vi "VI Tree.vi"   [LabVIEW 2021, in "Keysight XSAnVMA.lvlib"]
doc: "The VI Tree displays all the user-callable VIs of the instrument driver in an organized table."
uses:
  <instrlib>/Keysight XSAnVMA/Keysight XSAnVMA.lvlib
panel:
  # "XSAnVMA"
  # "1.0.4"
  # "SEE DIAGRAM\nFOR VI Tree"
  # "© Keysight Technologies 2018 - 2019"
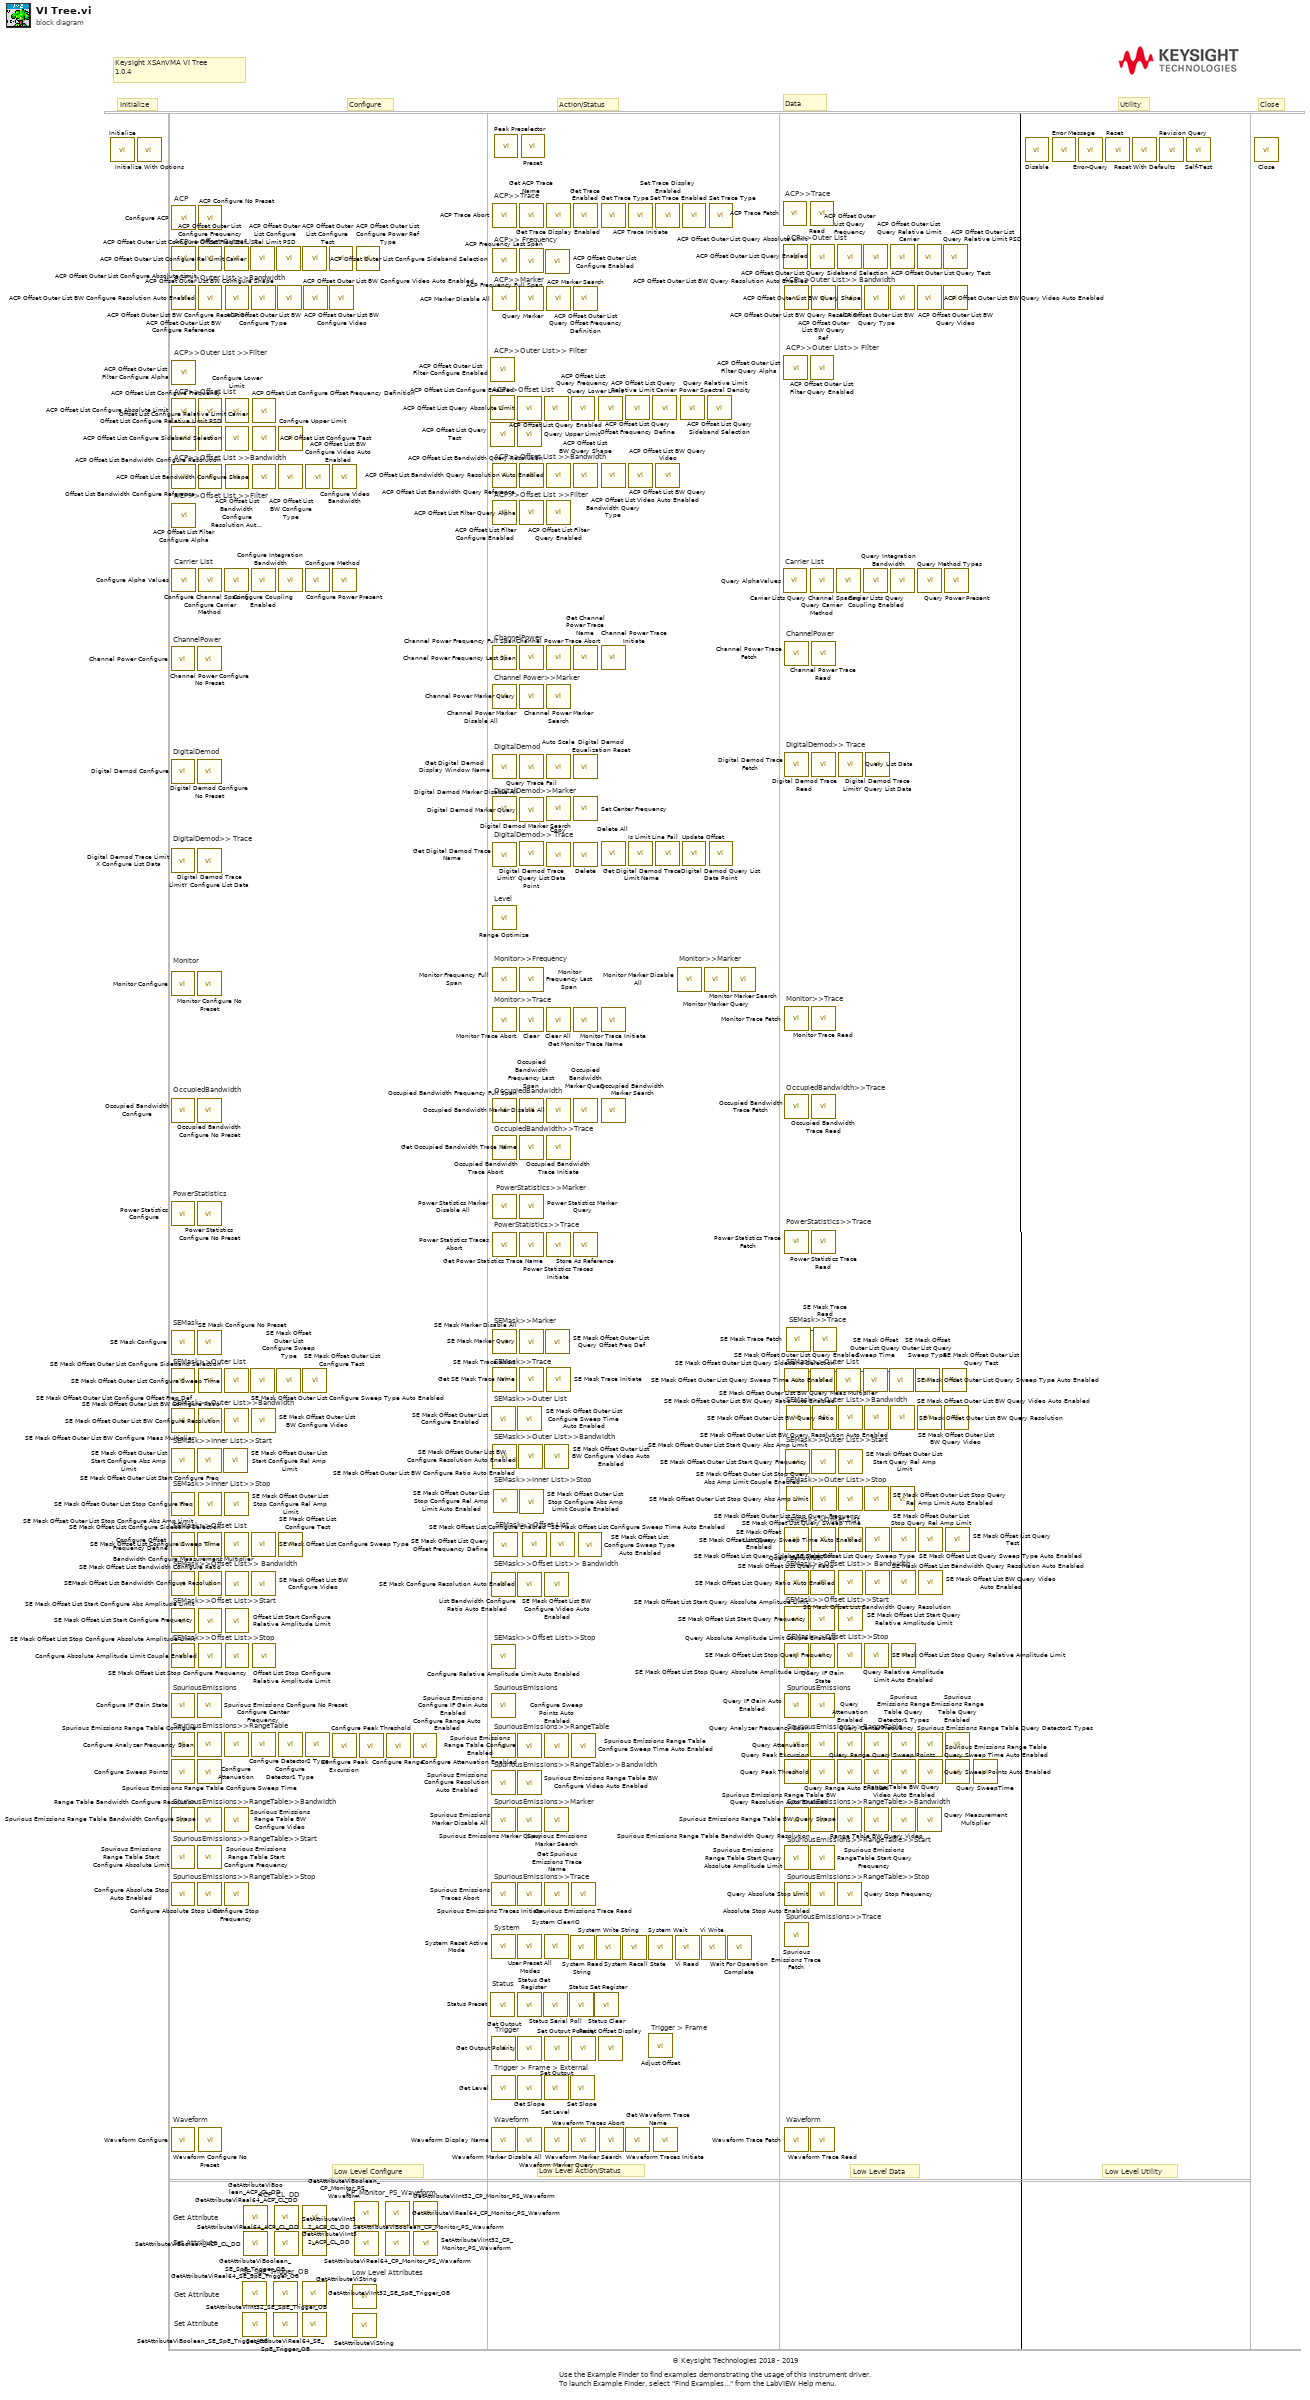
[diagram p0: block diagram]
diagram:
  # "Status"
  # "ACP>>Outer List"
  # "ACP>>Outer List>> Filter"
  # "ACP>>Outer List>> Bandwidth"
  # "Trigger > Frame > External"
  # "Trigger > Frame"
  # "Low Level Attributes"
  # "SE_SpE_Trigger_OB"
  # "CP_Monitor_PS_Waveform"
  # "Set Attribute"
  # "Get Attribute"
  # "Set Attribute"
  # "Get Attribute"
  # "ACP_CL_DD"
  # "Waveform"
  # "SpuriousEmissions>>Trace"
  # "SpuriousEmissions>>RangeTable>>Stop"
  # "SEMask>>Trace"
  # "ACP>>Trace"
  # "SpuriousEmissions>>RangeTable>>Bandwidth"
  # "SpuriousEmissions>>RangeTable"
  # "SpuriousEmissions"
  # "SEMask>>Offset List>>Stop"
  # "SEMask>>Offset List>> Bandwidth"
  # "SEMask>>Inner List>>Stop"
  # "SEMask>>Outer List>>Bandwidth"
  # "SEMask>>Outer List"
  # "ACP>>Offset Outer List"
  # "Waveform"
  # "SpuriousEmissions>>Trace"
  # "SpuriousEmissions>>RangeTable>>Stop"
  # "SpuriousEmissions>>RangeTable>>Start"
  # "SpuriousEmissions>>RangeTable>>Start"
  # "SpuriousEmissions>>RangeTable>>Bandwidth"
  # "SpuriousEmissions>>RangeTable>>Bandwidth"
  # "SpuriousEmissions>>RangeTable"
  # "SpuriousEmissions>>RangeTable"
  # "SpuriousEmissions"
  # "SpuriousEmissions>>Marker"
  # "SEMask>>Offset List"
  # "SEMask>>Trace"
  # "SEMask>>Outer List"
  # "SEMask>>Offset List>> Bandwidth"
  # "SEMask>>Offset List>>Stop"
  # "SEMask>>Offset List>>Start"
  # "SEMask>>Offset List>>Stop"
  # "SEMask>>Offset List>>Start"
  # "SEMask>>Offset List>> Bandwidth"
  # "SEMask>>Offset List"
  # "SEMask>>Offset List"
  # "SEMask>>Outer List>>Stop"
  # "SEMask>>Inner List>>Stop"
  # "SEMask>>Outer List>>Start"
  # "SEMask>>Inner List>>Start"
  # "SEMask>>Outer List>>Bandwidth"
  # "SEMask>>Outer List>>Bandwidth"
  # "SEMask>>Outer List"
  # "SEMask>>Marker"
  # "ChannelPower"
  # "Monitor>>Trace"
  # "OccupiedBandwidth>>Trace"
  # "PowerStatistics>>Trace"
  # "PowerStatistics>>Trace"
  # "PowerStatistics>>Marker"
  # "OccupiedBandwidth>>Trace"
  # "OccupiedBandwidth"
  # "Monitor>>Trace"
  # "Monitor>>Marker"
  # "Monitor>>Frequency"
  # "DigitalDemod>> Trace"
  # "DigitalDemod>> Trace"
  # "DigitalDemod>> Trace"
  # "DigitalDemod"
  # "ChannelPower"
  # "ACP>>Offset List >>Filter"
  # "ACP>>Outer List>> Filter"
  # "ACP>>Offset List >>Bandwidth"
  # "ACP>>Offset List"
  # "ACP>>Outer List >>Filter"
  # "ACP>>Outer List >>Bandwidth"
  # "ACP>> Frequency"
  # "Carrier List"
  # "Low Level Utility"
  # "Low Level Configure"
  # "Low Level Action/Status"
  # "Low Level Data"
  # "Action/Status"
  # "Keysight XSAnVMA VI Tree\n1.0.4"
  # "© Keysight Technologies 2018 - 2019"
  # "Close"
  # "Utility"
  # "Data"
  # "Configure"
  # "Initialize"
  # "Use the Example Finder to find examples demonstrating the usage of this instrument driver.\nTo launch Example Finder, select \"Find Examples...\" from the LabVIEW Help menu."
  # "Waveform"
  # "Trigger"
  # "System"
  # "SpuriousEmissions"
  # "SEMask"
  # "PowerStatistics"
  # "OccupiedBandwidth"
  # "Monitor"
  # "Level"
  # "DigitalDemod>>Marker"
  # "DigitalDemod"
  # "Channel Power>>Marker"
  # "ChannelPower"
  # "ACP>>Trace"
  # "ACP>>Offset List >>Filter"
  # "ACP>>Offset List >>Bandwidth"
  # "ACP>>Offset List"
  # "ACP>>Marker"
  # "Carrier List"
  # "ACP"
  n1 = call <instrlib>:"Initialize.vi"() -> ()  [unwired: 10 in, 2 out]
  n2 = call <instrlib>:"Initialize With Options.vi"() -> ()  [unwired: 10 in, 2 out]
  n3 = call <instrlib>:"Channel Power Configure.vi"() -> ()  [unwired: 10 in, 2 out]
  n4 = call <instrlib>:"Digital Demod Configure.vi"() -> ()  [unwired: 10 in, 2 out]
  n5 = call <instrlib>:"Digital Demod Trace Limit X Configure List Data.vi"() -> ()  [unwired: 10 in, 2 out]
  n6 = call <instrlib>:"Monitor Configure.vi"() -> ()  [unwired: 10 in, 2 out]
  n7 = call <instrlib>:"Occupied Bandwidth Configure.vi"() -> ()  [unwired: 10 in, 2 out]
  n8 = call <instrlib>:"Power Statistics Configure.vi"() -> ()  [unwired: 10 in, 2 out]
  n9 = call <instrlib>:"SE Mask Configure.vi"() -> ()  [unwired: 10 in, 2 out]
  n10 = call <instrlib>:"SE Mask Offset Outer List Configure Offset Freq Def.vi"() -> ()  [unwired: 10 in, 2 out]
  n11 = call <instrlib>:"SE Mask Offset Outer List BW Configure Meas Multiplier.vi"() -> ()  [unwired: 10 in, 2 out]
  n12 = call <instrlib>:"SE Mask Offset Outer List Start Configure Abs Amp Limit.vi"() -> ()  [unwired: 10 in, 2 out]
  n13 = call <instrlib>:"SE Mask Offset Outer List Stop Configure Abs Amp Limit.vi"() -> ()  [unwired: 10 in, 2 out]
  n14 = call <instrlib>:"Configure Offset Frequency Define.vi"() -> ()  [unwired: 10 in, 2 out]
  n15 = call <instrlib>:"Bandwidth Configure Measurement Multiplier.vi"() -> ()  [unwired: 10 in, 2 out]
  n16 = call <instrlib>:"SE Mask Offset List Start Configure Abs Amplitude Limit.vi"() -> ()  [unwired: 10 in, 2 out]
  n17 = call <instrlib>:"SE Mask Offset List Stop Configure Absolute Amplitude Limit.vi"() -> ()  [unwired: 10 in, 2 out]
  n18 = call <instrlib>:"Configure IF Gain State.vi"() -> ()  [unwired: 10 in, 2 out]
  n19 = call <instrlib>:"Spurious Emissions Range Table Configure.vi"() -> ()  [unwired: 10 in, 2 out]
  n20 = call <instrlib>:"Configure Sweep Points.vi"() -> ()  [unwired: 10 in, 2 out]
  n21 = call <instrlib>:"Range Table Bandwidth Configure Resolution.vi"() -> ()  [unwired: 10 in, 2 out]
  n22 = call <instrlib>:"Spurious Emissions Range Table Start Configure Absolute Limit.vi"() -> ()  [unwired: 10 in, 2 out]
  n23 = call <instrlib>:"Configure Absolute Stop Auto Enabled.vi"() -> ()  [unwired: 10 in, 2 out]
  n24 = call <instrlib>:"Waveform Configure.vi"() -> ()  [unwired: 10 in, 2 out]
  n25 = call <instrlib>:"Configure ACP.vi"() -> ()  [unwired: 10 in, 2 out]
  n26 = call <instrlib>:"ACP Offset Outer List Configure Absolute Limit.vi"() -> ()  [unwired: 10 in, 2 out]
  n27 = call <instrlib>:"ACP Offset Outer List BW Configure Reference.vi"() -> ()  [unwired: 10 in, 2 out]
  n28 = call <instrlib>:"ACP Offset Outer List Filter Configure Alpha.vi"() -> ()  [unwired: 10 in, 2 out]
  n29 = call <instrlib>:"ACP Offset List Configure Absolute Limit.vi"() -> ()  [unwired: 10 in, 2 out]
  n30 = call <instrlib>:"Offset List Configure Relative Limit Carrier.vi"() -> ()  [unwired: 10 in, 2 out]
  n31 = call <instrlib>:"Offset List Bandwidth Configure Reference.vi"() -> ()  [unwired: 10 in, 2 out]
  n32 = call <instrlib>:"ACP Offset List Filter Configure Alpha.vi"() -> ()  [unwired: 10 in, 2 out]
  n33 = call <instrlib>:"Configure Alpha Values.vi"() -> ()  [unwired: 10 in, 2 out]
  n34 = call <instrlib>:"Channel Power Configure No Preset.vi"() -> ()  [unwired: 10 in, 2 out]
  n35 = call <instrlib>:"Digital Demod Configure No Preset.vi"() -> ()  [unwired: 10 in, 2 out]
  n36 = call <instrlib>:"Digital Demod Trace LimitY Configure List Data.vi"() -> ()  [unwired: 10 in, 2 out]
  n37 = call <instrlib>:"Monitor Configure No Preset.vi"() -> ()  [unwired: 10 in, 2 out]
  n38 = call <instrlib>:"Occupied Bandwidth Configure No Preset.vi"() -> ()  [unwired: 10 in, 2 out]
  n39 = call <instrlib>:"Power Statistics Configure No Preset.vi"() -> ()  [unwired: 10 in, 2 out]
  n40 = call <instrlib>:"SE Mask Configure No Preset.vi"() -> ()  [unwired: 10 in, 2 out]
  n41 = call <instrlib>:"SE Mask Offset Outer List Start Configure Freq.vi"() -> ()  [unwired: 10 in, 2 out]
  n42 = call <instrlib>:"SE Mask Offset List Configure Sideband Selection.vi"() -> ()  [unwired: 10 in, 2 out]
  n43 = call <instrlib>:"Spurious Emissions Configure No Preset.vi"() -> ()  [unwired: 10 in, 2 out]
  n44 = call <instrlib>:"Configure Analyzer Frequency Span.vi"() -> ()  [unwired: 10 in, 2 out]
  n45 = call <instrlib>:"Spurious Emissions Range Table Configure Sweep Time.vi"() -> ()  [unwired: 10 in, 2 out]
  n46 = call <instrlib>:"Spurious Emissions Range Table Bandwidth Configure Shape.vi"() -> ()  [unwired: 10 in, 2 out]
  n47 = call <instrlib>:"Spurious Emissions Range Table Start Configure Frequency.vi"() -> ()  [unwired: 10 in, 2 out]
  n48 = call <instrlib>:"Configure Absolute Stop Limit.vi"() -> ()  [unwired: 10 in, 2 out]
  n49 = call <instrlib>:"ACP Configure No Preset.vi"() -> ()  [unwired: 10 in, 2 out]
  n50 = call <instrlib>:"ACP Offset Outer List Configure Frequency.vi"() -> ()  [unwired: 10 in, 2 out]
  n51 = call <instrlib>:"ACP Offset Outer List BW Configure Resolution Auto Enabled.vi"() -> ()  [unwired: 10 in, 2 out]
  n52 = call <instrlib>:"ACP Offset List Configure Frequency.vi"() -> ()  [unwired: 10 in, 2 out]
  n53 = call <instrlib>:"Offset List Configure Relative Limit PSD.vi"() -> ()  [unwired: 10 in, 2 out]
  n54 = call <instrlib>:"ACP Offset List Bandwidth Configure Resolution.vi"() -> ()  [unwired: 10 in, 2 out]
  n55 = call <instrlib>:"Configure Carrier Method.vi"() -> ()  [unwired: 10 in, 2 out]
  n56 = call <instrlib>:"SE Mask Offset Outer List Configure Sideband Selection.vi"() -> ()  [unwired: 10 in, 2 out]
  n57 = call <instrlib>:"SE Mask Offset Outer List BW Configure Ratio.vi"() -> ()  [unwired: 10 in, 2 out]
  n58 = call <instrlib>:"SE Mask Offset Outer List Stop Configure Freq.vi"() -> ()  [unwired: 10 in, 2 out]
  n59 = call <instrlib>:"SE Mask Offset List Bandwidth Configure Ratio.vi"() -> ()  [unwired: 10 in, 2 out]
  n60 = call <instrlib>:"SE Mask Offset List Start Configure Frequency.vi"() -> ()  [unwired: 10 in, 2 out]
  n61 = call <instrlib>:"Configure Absolute Amplitude Limit Couple Enabled.vi"() -> ()  [unwired: 10 in, 2 out]
  n62 = call <instrlib>:"Waveform Configure No Preset.vi"() -> ()  [unwired: 10 in, 2 out]
  n63 = call <instrlib>:"SE Mask Offset Outer List Start Configure Rel Amp Limit.vi"() -> ()  [unwired: 10 in, 2 out]
  n64 = call <instrlib>:"ACP Offset Outer List Configure Offset Freq Def.vi"() -> ()  [unwired: 10 in, 2 out]
  n65 = call <instrlib>:"Configure Channel Spacing.vi"() -> ()  [unwired: 10 in, 2 out]
  n66 = call <instrlib>:"SE Mask Offset Outer List Configure Sweep Time.vi"() -> ()  [unwired: 10 in, 2 out]
  n67 = call <instrlib>:"SE Mask Offset Outer List BW Configure Resolution.vi"() -> ()  [unwired: 10 in, 2 out]
  n68 = call <instrlib>:"SE Mask Offset Outer List Stop Configure Rel Amp Limit.vi"() -> ()  [unwired: 10 in, 2 out]
  n69 = call <instrlib>:"SE Mask Offset List Configure Sweep Time.vi"() -> ()  [unwired: 10 in, 2 out]
  n70 = call <instrlib>:"Configure Attenuation.vi"() -> ()  [unwired: 10 in, 2 out]
  n71 = call <instrlib>:"Spurious Emissions Range Table BW Configure Video.vi"() -> ()  [unwired: 10 in, 2 out]
  n72 = call <instrlib>:"Configure Stop Frequency.vi"() -> ()  [unwired: 10 in, 2 out]
  n73 = call <instrlib>:"ACP Offset Outer List BW Configure Resolution.vi"() -> ()  [unwired: 10 in, 2 out]
  n74 = call <instrlib>:"Configure Lower Limit.vi"() -> ()  [unwired: 10 in, 2 out]
  n75 = call <instrlib>:"ACP Offset List Configure Sideband Selection.vi"() -> ()  [unwired: 10 in, 2 out]
  n76 = call <instrlib>:"ACP Offset List Bandwidth Configure Resolution Auto Enabled.vi"() -> ()  [unwired: 10 in, 2 out]
  n77 = call <instrlib>:"SEMask Offset List Bandwidth Configure Resolution.vi"() -> ()  [unwired: 10 in, 2 out]
  n78 = call <instrlib>:"Offset List Start Configure Relative Amplitude Limit.vi"() -> ()  [unwired: 10 in, 2 out]
  n79 = call <instrlib>:"SE Mask Offset List Stop Configure Frequency.vi"() -> ()  [unwired: 10 in, 2 out]
  n80 = call <instrlib>:"GetAttributeViBoolean_SE_SpE_Trigger_OB.vi"() -> ()  [unwired: 9 in, 3 out]
  n81 = call <instrlib>:"SetAttributeViBoolean_SE_SpE_Trigger_OB.vi"() -> ()  [unwired: 10 in, 2 out]
  n82 = call <instrlib>:"GetAttributeViBoolean_ACP_CL_DD.vi"() -> ()  [unwired: 9 in, 3 out]
  n83 = call <instrlib>:"SetAttributeViBoolean_ACP_CL_DD.vi"() -> ()  [unwired: 10 in, 2 out]
  n84 = call <instrlib>:"ACP Offset Outer List Configure Rel Limit Carrier.vi"() -> ()  [unwired: 10 in, 2 out]
  n85 = call <instrlib>:"SE Mask Offset Outer List Configure Sweep Type Auto Enabled.vi"() -> ()  [unwired: 10 in, 2 out]
  n86 = call <instrlib>:"ACP Offset Outer List BW Configure Shape.vi"() -> ()  [unwired: 10 in, 2 out]
  n87 = call <instrlib>:"Configure Coupling Enabled.vi"() -> ()  [unwired: 10 in, 2 out]
  n88 = call <instrlib>:"SE Mask Offset Outer List BW Configure Video.vi"() -> ()  [unwired: 10 in, 2 out]
  n89 = call <instrlib>:"SE Mask Offset List Configure Sweep Type.vi"() -> ()  [unwired: 10 in, 2 out]
  n90 = call <instrlib>:"SE Mask Offset List BW Configure Video.vi"() -> ()  [unwired: 10 in, 2 out]
  n91 = call <instrlib>:"Configure Center Frequency.vi"() -> ()  [unwired: 10 in, 2 out]
  n92 = call <instrlib>:"ACP Offset List Configure Offset Frequency Definition.vi"() -> ()  [unwired: 10 in, 2 out]
  n93 = call <instrlib>:"ACP Offset List Configure Test.vi"() -> ()  [unwired: 10 in, 2 out]
  n94 = call <instrlib>:"ACP Offset List Bandwidth Configure Shape.vi"() -> ()  [unwired: 10 in, 2 out]
  n95 = call <instrlib>:"Offset List Stop Configure Relative Amplitude Limit.vi"() -> ()  [unwired: 10 in, 2 out]
  n96 = call <instrlib>:"GetAttributeViReal64_SE_SpE_Trigger_OB.vi"() -> ()  [unwired: 9 in, 3 out]
  n97 = call <instrlib>:"SetAttributeViReal64_SE_SpE_Trigger_OB.vi"() -> ()  [unwired: 10 in, 2 out]
  n98 = call <instrlib>:"GetAttributeViReal64_ACP_CL_DD.vi"() -> ()  [unwired: 9 in, 3 out]
  n99 = call <instrlib>:"SetAttributeViReal64_ACP_CL_DD.vi"() -> ()  [unwired: 10 in, 2 out]
  n100 = call <instrlib>:"ACP Offset Outer List Configure Rel Limit PSD.vi"() -> ()  [unwired: 10 in, 2 out]
  n101 = call <instrlib>:"SE Mask Offset Outer List Configure Sweep Type.vi"() -> ()  [unwired: 10 in, 2 out]
  n102 = call <instrlib>:"ACP Offset Outer List BW Configure Type.vi"() -> ()  [unwired: 10 in, 2 out]
  n103 = call <instrlib>:"Configure Integration Bandwidth.vi"() -> ()  [unwired: 10 in, 2 out]
  n104 = call <instrlib>:"SE Mask Offset List Configure Test.vi"() -> ()  [unwired: 10 in, 2 out]
  n105 = call <instrlib>:"Configure Detector1 Type.vi"() -> ()  [unwired: 10 in, 2 out]
  n106 = call <instrlib>:"Configure Upper Limit.vi"() -> ()  [unwired: 10 in, 2 out]
  n107 = call <instrlib>:"ACP Offset List BW Configure Type.vi"() -> ()  [unwired: 10 in, 2 out]
  n108 = call <instrlib>:"GetAttributeViInt32_SE_SpE_Trigger_OB.vi"() -> ()  [unwired: 9 in, 3 out]
  n109 = call <instrlib>:"SetAttributeViInt32_SE_SpE_Trigger_OB.vi"() -> ()  [unwired: 10 in, 2 out]
  n110 = call <instrlib>:"ACP Offset Outer List Configure Sideband Selection.vi"() -> ()  [unwired: 10 in, 2 out]
  n111 = call <instrlib>:"SE Mask Offset Outer List Configure Test.vi"() -> ()  [unwired: 10 in, 2 out]
  n112 = call <instrlib>:"GetAttributeViInt32_ACP_CL_DD.vi"() -> ()  [unwired: 9 in, 3 out]
  n113 = call <instrlib>:"SetAttributeViInt32_ACP_CL_DD.vi"() -> ()  [unwired: 10 in, 2 out]
  n114 = call <instrlib>:"ACP Offset Outer List BW Configure Video Auto Enabled.vi"() -> ()  [unwired: 10 in, 2 out]
  n115 = call <instrlib>:"Configure Method.vi"() -> ()  [unwired: 10 in, 2 out]
  n116 = call <instrlib>:"Configure Detector2 Type.vi"() -> ()  [unwired: 10 in, 2 out]
  n117 = call <instrlib>:"ACP Offset List BW Configure Video Auto Enabled.vi"() -> ()  [unwired: 10 in, 2 out]
  n118 = call <instrlib>:"ACP Offset Outer List Configure Test.vi"() -> ()  [unwired: 10 in, 2 out]
  n119 = call <instrlib>:"ACP Offset Outer List BW Configure Video.vi"() -> ()  [unwired: 10 in, 2 out]
  n120 = call <instrlib>:"Configure Power Present.vi"() -> ()  [unwired: 10 in, 2 out]
  n121 = call <instrlib>:"Configure Peak Excursion.vi"() -> ()  [unwired: 10 in, 2 out]
  n122 = call <instrlib>:"Configure Video Bandwidth.vi"() -> ()  [unwired: 10 in, 2 out]
  n123 = call <instrlib>:"GetAttributeViString.vi"() -> ()  [unwired: 9 in, 3 out]
  n124 = call <instrlib>:"SetAttributeViString.vi"() -> ()  [unwired: 10 in, 2 out]
  n125 = call <instrlib>:"GetAttributeViBoolean_CP_Monitor_PS_Waveform.vi"() -> ()  [unwired: 9 in, 3 out]
  n126 = call <instrlib>:"SetAttributeViBoolean_CP_Monitor_PS_Waveform.vi"() -> ()  [unwired: 10 in, 2 out]
  n127 = call <instrlib>:"ACP Offset Outer List Configure Power Ref Type.vi"() -> ()  [unwired: 10 in, 2 out]
  n128 = call <instrlib>:"Configure Peak Threshold.vi"() -> ()  [unwired: 10 in, 2 out]
  n129 = call <instrlib>:"GetAttributeViReal64_CP_Monitor_PS_Waveform.vi"() -> ()  [unwired: 9 in, 3 out]
  n130 = call <instrlib>:"SetAttributeViReal64_CP_Monitor_PS_Waveform.vi"() -> ()  [unwired: 10 in, 2 out]
  n131 = call <instrlib>:"Configure Range.vi"() -> ()  [unwired: 10 in, 2 out]
  n132 = call <instrlib>:"Configure Range Auto Enabled.vi"() -> ()  [unwired: 10 in, 2 out]
  n133 = call <instrlib>:"GetAttributeViInt32_CP_Monitor_PS_Waveform.vi"() -> ()  [unwired: 9 in, 3 out]
  n134 = call <instrlib>:"SetAttributeViInt32_CP_Monitor_PS_Waveform.vi"() -> ()  [unwired: 10 in, 2 out]
  n135 = call <instrlib>:"ACP Offset List Configure Enabled.vi"() -> ()  [unwired: 10 in, 2 out]
  n136 = call <instrlib>:"ACP Offset Outer List Filter Configure Enabled.vi"() -> ()  [unwired: 10 in, 2 out]
  n137 = call <instrlib>:"ACP Offset List Query Test.vi"() -> ()  [unwired: 8 in, 4 out]
  n138 = call <instrlib>:"Status Preset.vi"() -> ()  [unwired: 10 in, 2 out]
  n139 = call <instrlib>:"SE Mask Offset Outer List Configure Enabled.vi"() -> ()  [unwired: 10 in, 2 out]
  n140 = call <instrlib>:"List Bandwidth Configure Ratio Auto Enabled.vi"() -> ()  [unwired: 10 in, 2 out]
  n141 = call <instrlib>:"Configure Relative Amplitude Limit Auto Enabled.vi"() -> ()  [unwired: 10 in, 2 out]
  n142 = call <instrlib>:"Spurious Emissions Configure IF Gain Auto Enabled.vi"() -> ()  [unwired: 10 in, 2 out]
  n143 = call <instrlib>:"Configure Attenuation Enabled.vi"() -> ()  [unwired: 10 in, 2 out]
  n144 = call <instrlib>:"Spurious Emissions Configure Resolution Auto Enabled.vi"() -> ()  [unwired: 10 in, 2 out]
  n145 = call <instrlib>:"Spurious Emissions Marker Disable All.vi"() -> ()  [unwired: 10 in, 2 out]
  n146 = call <instrlib>:"Spurious Emissions Traces Abort.vi"() -> ()  [unwired: 10 in, 2 out]
  n147 = call <instrlib>:"System Reset Active Mode.vi"() -> ()  [unwired: 10 in, 2 out]
  n148 = call <instrlib>:"Get Output.vi"() -> ()  [unwired: 9 in, 3 out]
  n149 = call <instrlib>:"Get Level.vi"() -> ()  [unwired: 9 in, 3 out]
  n150 = call <instrlib>:"Waveform Display Name.vi"() -> ()  [unwired: 9 in, 3 out]
  n151 = call <instrlib>:"ACP Trace Abort.vi"() -> ()  [unwired: 10 in, 2 out]
  n152 = call <instrlib>:"ACP Frequency Full Span.vi"() -> ()  [unwired: 10 in, 2 out]
  n153 = call <instrlib>:"ACP Marker Disable All.vi"() -> ()  [unwired: 10 in, 2 out]
  n154 = call <instrlib>:"ACP Offset List Bandwidth Query Reference.vi"() -> ()  [unwired: 8 in, 4 out]
  n155 = call <instrlib>:"ACP Offset List Filter Configure Enabled.vi"() -> ()  [unwired: 10 in, 2 out]
  n156 = call <instrlib>:"Channel Power Frequency Full Span.vi"() -> ()  [unwired: 10 in, 2 out]
  n157 = call <instrlib>:"Channel Power Marker Disable All.vi"() -> ()  [unwired: 10 in, 2 out]
  n158 = call <instrlib>:"Get Digital Demod Display Window Name.vi"() -> ()  [unwired: 9 in, 3 out]
  n159 = call <instrlib>:"Digital Demod Marker Disable All.vi"() -> ()  [unwired: 10 in, 2 out]
  n160 = call <instrlib>:"Get Digital Demod Trace Name.vi"() -> ()  [unwired: 9 in, 3 out]
  n161 = call <instrlib>:"Range Optimize.vi"() -> ()  [unwired: 10 in, 2 out]
  n162 = call <instrlib>:"Monitor Frequency Full Span.vi"() -> ()  [unwired: 10 in, 2 out]
  n163 = call <instrlib>:"Monitor Trace Abort.vi"() -> ()  [unwired: 10 in, 2 out]
  n164 = call <instrlib>:"Occupied Bandwidth Frequency Full Span.vi"() -> ()  [unwired: 10 in, 2 out]
  n165 = call <instrlib>:"Occupied Bandwidth Trace Abort.vi"() -> ()  [unwired: 10 in, 2 out]
  n166 = call <instrlib>:"Power Statistics Marker Disable All.vi"() -> ()  [unwired: 10 in, 2 out]
  n167 = call <instrlib>:"Power Statistics Traces Abort.vi"() -> ()  [unwired: 10 in, 2 out]
  n168 = call <instrlib>:"SE Mask Marker Disable All.vi"() -> ()  [unwired: 10 in, 2 out]
  n169 = call <instrlib>:"SE Mask Trace Abort.vi"() -> ()  [unwired: 10 in, 2 out]
  n170 = call <instrlib>:"SE Mask Offset Outer List BW Configure Ratio Auto Enabled.vi"() -> ()  [unwired: 10 in, 2 out]
  n171 = call <instrlib>:"SE Mask Offset Outer List Stop Configure Rel Amp Limit Auto Enabled.vi"() -> ()  [unwired: 10 in, 2 out]
  n172 = call <instrlib>:"SE Mask Offset List Query Offset Frequency Define.vi"() -> ()  [unwired: 9 in, 3 out]
  n173 = call <instrlib>:"Peak Preselector.vi"() -> ()  [unwired: 10 in, 2 out]
  n174 = call <instrlib>:"ACP Offset List Query Absolute Limit.vi"() -> ()  [unwired: 8 in, 4 out]
  n175 = call <instrlib>:"Query Upper Limit.vi"() -> ()  [unwired: 8 in, 4 out]
  n176 = call <instrlib>:"SE Mask Offset Outer List Configure Sweep Time Auto Enabled.vi"() -> ()  [unwired: 10 in, 2 out]
  n177 = call <instrlib>:"SE Mask Configure Resolution Auto Enabled.vi"() -> ()  [unwired: 10 in, 2 out]
  n178 = call <instrlib>:"Spurious Emissions Range Table Configure Enabled.vi"() -> ()  [unwired: 10 in, 2 out]
  n179 = call <instrlib>:"Spurious Emissions Range Table BW Configure Video Auto Enabled.vi"() -> ()  [unwired: 10 in, 2 out]
  n180 = call <instrlib>:"Spurious Emissions Marker Query.vi"() -> ()  [unwired: 8 in, 4 out]
  n181 = call <instrlib>:"Spurious Emissions Traces Initiate.vi"() -> ()  [unwired: 10 in, 2 out]
  n182 = call <instrlib>:"User Preset All Modes.vi"() -> ()  [unwired: 10 in, 2 out]
  n183 = call <instrlib>:"Status Get Register.vi"() -> ()  [unwired: 9 in, 3 out]
  n184 = call <instrlib>:"Get Output Polarity.vi"() -> ()  [unwired: 9 in, 3 out]
  n185 = call <instrlib>:"Get Slope.vi"() -> ()  [unwired: 9 in, 3 out]
  n186 = call <instrlib>:"Waveform Marker Disable All.vi"() -> ()  [unwired: 10 in, 2 out]
  n187 = call <instrlib>:"SE Mask Offset Outer List BW Configure Resolution Auto Enabled.vi"() -> ()  [unwired: 10 in, 2 out]
  n188 = call <instrlib>:"Get ACP Trace Name.vi"() -> ()  [unwired: 9 in, 3 out]
  n189 = call <instrlib>:"ACP Frequency Last Span.vi"() -> ()  [unwired: 10 in, 2 out]
  n190 = call <instrlib>:"Query Marker.vi"() -> ()  [unwired: 8 in, 4 out]
  n191 = call <instrlib>:"ACP Offset List Bandwidth Query Resolution.vi"() -> ()  [unwired: 8 in, 4 out]
  n192 = call <instrlib>:"ACP Offset List Filter Query Alpha.vi"() -> ()  [unwired: 8 in, 4 out]
  n193 = call <instrlib>:"Channel Power Frequency Last Span.vi"() -> ()  [unwired: 10 in, 2 out]
  n194 = call <instrlib>:"Channel Power Marker Query.vi"() -> ()  [unwired: 8 in, 4 out]
  n195 = call <instrlib>:"Query Trace Fail.vi"() -> ()  [unwired: 9 in, 3 out]
  n196 = call <instrlib>:"Digital Demod Marker Query.vi"() -> ()  [unwired: 8 in, 4 out]
  n197 = call <instrlib>:"Digital Demod Trace LimitY Query List Data Point.vi"() -> ()  [unwired: 9 in, 3 out]
  n198 = call <instrlib>:"Monitor Frequency Last Span.vi"() -> ()  [unwired: 10 in, 2 out]
  n199 = call <instrlib>:"Clear.vi"() -> ()  [unwired: 10 in, 2 out]
  n200 = call <instrlib>:"Occupied Bandwidth Frequency Last Span.vi"() -> ()  [unwired: 10 in, 2 out]
  n201 = call <instrlib>:"Get Occupied Bandwidth Trace Name.vi"() -> ()  [unwired: 9 in, 3 out]
  n202 = call <instrlib>:"Power Statistics Marker Query.vi"() -> ()  [unwired: 8 in, 4 out]
  n203 = call <instrlib>:"Get Power Statistics Trace Name.vi"() -> ()  [unwired: 9 in, 3 out]
  n204 = call <instrlib>:"SE Mask Marker Query.vi"() -> ()  [unwired: 8 in, 4 out]
  n205 = call <instrlib>:"Get SE Mask Trace Name.vi"() -> ()  [unwired: 9 in, 3 out]
  n206 = call <instrlib>:"SE Mask Offset Outer List Stop Configure Abs Amp Limit Couple Enabled.vi"() -> ()  [unwired: 10 in, 2 out]
  n207 = call <instrlib>:"Preset.vi"() -> ()  [unwired: 10 in, 2 out]
  n208 = call <instrlib>:"SE Mask Offset List Configure Enabled.vi"() -> ()  [unwired: 10 in, 2 out]
  n209 = call <instrlib>:"Status Serial Poll.vi"() -> ()  [unwired: 9 in, 3 out]
  n210 = call <instrlib>:"ACP Offset List Query Enabled.vi"() -> ()  [unwired: 8 in, 4 out]
  n211 = call <instrlib>:"System ClearIO.vi"() -> ()  [unwired: 10 in, 2 out]
  n212 = call <instrlib>:"Set Level.vi"() -> ()  [unwired: 10 in, 2 out]
  n213 = call <instrlib>:"SE Mask Offset Outer List BW Configure Video Auto Enabled.vi"() -> ()  [unwired: 10 in, 2 out]
  n214 = call <instrlib>:"SE Mask Offset List BW Configure Video Auto Enabled.vi"() -> ()  [unwired: 10 in, 2 out]
  n215 = call <instrlib>:"Configure Sweep Points Auto Enabled.vi"() -> ()  [unwired: 10 in, 2 out]
  n216 = call <instrlib>:"Spurious Emissions Marker Search.vi"() -> ()  [unwired: 10 in, 2 out]
  n217 = call <instrlib>:"Get Spurious Emissions Trace Name.vi"() -> ()  [unwired: 9 in, 3 out]
  n218 = call <instrlib>:"Set Output.vi"() -> ()  [unwired: 10 in, 2 out]
  n219 = call <instrlib>:"Waveform Marker Query.vi"() -> ()  [unwired: 8 in, 4 out]
  n220 = call <instrlib>:"ACP Offset Outer List Configure Enabled.vi"() -> ()  [unwired: 10 in, 2 out]
  n221 = call <instrlib>:"SE Mask Offset Outer List Query Offset Freq Def.vi"() -> ()  [unwired: 9 in, 3 out]
  n222 = call <instrlib>:"Get Trace Display Enabled.vi"() -> ()  [unwired: 9 in, 3 out]
  n223 = call <instrlib>:"ACP Marker Search.vi"() -> ()  [unwired: 10 in, 2 out]
  n224 = call <instrlib>:"ACP Offset List Bandwidth Query Resolution Auto Enabled.vi"() -> ()  [unwired: 8 in, 4 out]
  n225 = call <instrlib>:"ACP Offset List Filter Query Enabled.vi"() -> ()  [unwired: 8 in, 4 out]
  n226 = call <instrlib>:"Channel Power Trace Abort.vi"() -> ()  [unwired: 10 in, 2 out]
  n227 = call <instrlib>:"Channel Power Marker Search.vi"() -> ()  [unwired: 10 in, 2 out]
  n228 = call <instrlib>:"Auto Scale.vi"() -> ()  [unwired: 10 in, 2 out]
  n229 = call <instrlib>:"Digital Demod Marker Search.vi"() -> ()  [unwired: 10 in, 2 out]
  n230 = call <instrlib>:"Copy.vi"() -> ()  [unwired: 10 in, 2 out]
  n231 = call <instrlib>:"Clear All.vi"() -> ()  [unwired: 10 in, 2 out]
  n232 = call <instrlib>:"Occupied Bandwidth Marker Disable All.vi"() -> ()  [unwired: 10 in, 2 out]
  n233 = call <instrlib>:"Occupied Bandwidth Trace Initiate.vi"() -> ()  [unwired: 10 in, 2 out]
  n234 = call <instrlib>:"Power Statistics Traces Initiate.vi"() -> ()  [unwired: 10 in, 2 out]
  n235 = call <instrlib>:"SE Mask Trace Initiate.vi"() -> ()  [unwired: 10 in, 2 out]
  n236 = call <instrlib>:"SE Mask Offset List Configure Sweep Time Auto Enabled.vi"() -> ()  [unwired: 10 in, 2 out]
  n237 = call <instrlib>:"Status Set Register.vi"() -> ()  [unwired: 10 in, 2 out]
  n238 = call <instrlib>:"System Read String.vi"() -> ()  [unwired: 9 in, 3 out]
  n239 = call <instrlib>:"Set Slope.vi"() -> ()  [unwired: 10 in, 2 out]
  n240 = call <instrlib>:"ACP Offset List Query Frequency.vi"() -> ()  [unwired: 8 in, 4 out]
  n241 = call <instrlib>:"Spurious Emissions Range Table Configure Sweep Time Auto Enabled.vi"() -> ()  [unwired: 10 in, 2 out]
  n242 = call <instrlib>:"Spurious Emissions Trace Read.vi"() -> ()  [unwired: 8 in, 4 out]
  n243 = call <instrlib>:"Set Output Polarity.vi"() -> ()  [unwired: 10 in, 2 out]
  n244 = call <instrlib>:"Waveform Marker Search.vi"() -> ()  [unwired: 10 in, 2 out]
  n245 = call <instrlib>:"Get Trace Enabled.vi"() -> ()  [unwired: 9 in, 3 out]
  n246 = call <instrlib>:"ACP Offset Outer List Query Offset Frequency Definition.vi"() -> ()  [unwired: 9 in, 3 out]
  n247 = call <instrlib>:"ACP Offset List BW Query Shape.vi"() -> ()  [unwired: 8 in, 4 out]
  n248 = call <instrlib>:"Get Channel Power Trace Name.vi"() -> ()  [unwired: 9 in, 3 out]
  n249 = call <instrlib>:"Digital Demod Equalization Reset.vi"() -> ()  [unwired: 10 in, 2 out]
  n250 = call <instrlib>:"Set Center Frequency.vi"() -> ()  [unwired: 10 in, 2 out]
  n251 = call <instrlib>:"Delete.vi"() -> ()  [unwired: 10 in, 2 out]
  n252 = call <instrlib>:"Get Monitor Trace Name.vi"() -> ()  [unwired: 9 in, 3 out]
  n253 = call <instrlib>:"Occupied Bandwidth Marker Query.vi"() -> ()  [unwired: 8 in, 4 out]
  n254 = call <instrlib>:"Store As Reference.vi"() -> ()  [unwired: 10 in, 2 out]
  n255 = call <instrlib>:"SE Mask Offset List Configure Sweep Type Auto Enabled.vi"() -> ()  [unwired: 10 in, 2 out]
  n256 = call <instrlib>:"Status Clear.vi"() -> ()  [unwired: 10 in, 2 out]
  n257 = call <instrlib>:"System Write String.vi"() -> ()  [unwired: 10 in, 2 out]
  n258 = call <instrlib>:"Query Lower Limit.vi"() -> ()  [unwired: 8 in, 4 out]
  n259 = call <instrlib>:"Reset Offset Display.vi"() -> ()  [unwired: 10 in, 2 out]
  n260 = call <instrlib>:"Waveform Traces Abort.vi"() -> ()  [unwired: 10 in, 2 out]
  n261 = call <instrlib>:"Get Trace Type.vi"() -> ()  [unwired: 9 in, 3 out]
  n262 = call <instrlib>:"ACP Offset List Bandwidth Query Type.vi"() -> ()  [unwired: 8 in, 4 out]
  n263 = call <instrlib>:"Channel Power Trace Initiate.vi"() -> ()  [unwired: 10 in, 2 out]
  n264 = call <instrlib>:"Delete All.vi"() -> ()  [unwired: 10 in, 2 out]
  n265 = call <instrlib>:"Monitor Trace Initiate.vi"() -> ()  [unwired: 10 in, 2 out]
  n266 = call <instrlib>:"Occupied Bandwidth Marker Search.vi"() -> ()  [unwired: 10 in, 2 out]
  n267 = call <instrlib>:"System Recall State.vi"() -> ()  [unwired: 10 in, 2 out]
  n268 = call <instrlib>:"ACP Offset List Query Offset Frequency Define.vi"() -> ()  [unwired: 9 in, 3 out]
  n269 = call <instrlib>:"Get Waveform Trace Name.vi"() -> ()  [unwired: 9 in, 3 out]
  n270 = call <instrlib>:"ACP Trace Initiate.vi"() -> ()  [unwired: 10 in, 2 out]
  n271 = call <instrlib>:"ACP Offset List BW Query Video.vi"() -> ()  [unwired: 8 in, 4 out]
  n272 = call <instrlib>:"Is Limit Line Fail.vi"() -> ()  [unwired: 9 in, 3 out]
  n273 = call <instrlib>:"System Wait.vi"() -> ()  [unwired: 10 in, 2 out]
  n274 = call <instrlib>:"Adjust Offset.vi"() -> ()  [unwired: 10 in, 2 out]
  n275 = call <instrlib>:"ACP Offset List Query Relative Limit Carrier.vi"() -> ()  [unwired: 8 in, 4 out]
  n276 = call <instrlib>:"Waveform Traces Initiate.vi"() -> ()  [unwired: 10 in, 2 out]
  n277 = call <instrlib>:"Set Trace Display Enabled.vi"() -> ()  [unwired: 10 in, 2 out]
  n278 = call <instrlib>:"ACP Offset List BW Query Video Auto Enabled.vi"() -> ()  [unwired: 8 in, 4 out]
  n279 = call <instrlib>:"Get Digital Demod Trace Limit Name.vi"() -> ()  [unwired: 9 in, 3 out]
  n280 = call <instrlib>:"Vi Read.vi"() -> ()  [unwired: 8 in, 4 out]
  n281 = call <instrlib>:"Monitor Marker Disable All.vi"() -> ()  [unwired: 10 in, 2 out]
  n282 = call <instrlib>:"Query Relative Limit Power Spectral Density.vi"() -> ()  [unwired: 8 in, 4 out]
  n283 = call <instrlib>:"Set Trace Enabled.vi"() -> ()  [unwired: 10 in, 2 out]
  n284 = call <instrlib>:"Update Offset.vi"() -> ()  [unwired: 10 in, 2 out]
  n285 = call <instrlib>:"Vi Write.vi"() -> ()  [unwired: 9 in, 3 out]
  n286 = call <instrlib>:"Monitor Marker Query.vi"() -> ()  [unwired: 8 in, 4 out]
  n287 = call <instrlib>:"ACP Offset List Query Sideband Selection.vi"() -> ()  [unwired: 8 in, 4 out]
  n288 = call <instrlib>:"Set Trace Type.vi"() -> ()  [unwired: 10 in, 2 out]
  n289 = call <instrlib>:"Digital Demod Query List Data Point.vi"() -> ()  [unwired: 9 in, 3 out]
  n290 = call <instrlib>:"Wait For Operation Complete.vi"() -> ()  [unwired: 10 in, 2 out]
  n291 = call <instrlib>:"Monitor Marker Search.vi"() -> ()  [unwired: 10 in, 2 out]
  n292 = call <instrlib>:"ACP Trace Fetch.vi"() -> ()  [unwired: 8 in, 4 out]
  n293 = call <instrlib>:"Query AlphaValues.vi"() -> ()  [unwired: 8 in, 4 out]
  n294 = call <instrlib>:"ACP Offset Outer List Query Absolute Limit.vi"() -> ()  [unwired: 8 in, 4 out]
  n295 = call <instrlib>:"ACP Offset Outer List Filter Query Alpha.vi"() -> ()  [unwired: 8 in, 4 out]
  n296 = call <instrlib>:"ACP Offset Outer List BW Query Resolution Auto Enabled.vi"() -> ()  [unwired: 8 in, 4 out]
  n297 = call <instrlib>:"Channel Power Trace Fetch.vi"() -> ()  [unwired: 8 in, 4 out]
  n298 = call <instrlib>:"Digital Demod Trace Fetch.vi"() -> ()  [unwired: 8 in, 4 out]
  n299 = call <instrlib>:"Monitor Trace Fetch.vi"() -> ()  [unwired: 8 in, 4 out]
  n300 = call <instrlib>:"Occupied Bandwidth Trace Fetch.vi"() -> ()  [unwired: 8 in, 4 out]
  n301 = call <instrlib>:"Power Statistics Trace Fetch.vi"() -> ()  [unwired: 8 in, 4 out]
  n302 = call <instrlib>:"SE Mask Offset Outer List Query Enabled.vi"() -> ("instrument handle out"=w4:refnum<k15>)  [unwired: 8 in, 3 out]
  n303 = call <instrlib>:"SE Mask Offset List Query Enabled.vi"() -> ()  [unwired: 8 in, 4 out]
  n304 = call <instrlib>:"Query Bandwidth.vi"() -> ()  [unwired: 8 in, 4 out]
  n305 = call <instrlib>:"SE Mask Offset List Start Query Absolute Amplitude Limit.vi"() -> ()  [unwired: 8 in, 4 out]
  n306 = call <instrlib>:"SE Mask Offset List Stop Query Absolute Amplitude Limit.vi"() -> ()  [unwired: 8 in, 4 out]
  n307 = call <instrlib>:"Query IF Gain Auto Enabled.vi"() -> ()  [unwired: 8 in, 4 out]
  n308 = call <instrlib>:"Query Analyzer Frequency Span.vi"() -> ()  [unwired: 8 in, 4 out]
  n309 = call <instrlib>:"Query Peak Excursion.vi"() -> ()  [unwired: 8 in, 4 out]
  n310 = call <instrlib>:"Spurious Emissions Range Table Bandwidth Query Resolution.vi"() -> ()  [unwired: 8 in, 4 out]
  n311 = call <instrlib>:"Spurious Emissions Range Table Start Query Absolute Amplitude Limit.vi"() -> ()  [unwired: 8 in, 4 out]
  n312 = call <instrlib>:"Absolute Stop Auto Enabled.vi"() -> ()  [unwired: 8 in, 4 out]
  n313 = call <instrlib>:"Spurious Emissions Trace Fetch.vi"() -> ()  [unwired: 8 in, 4 out]
  n314 = call <instrlib>:"Waveform Trace Fetch.vi"() -> ()  [unwired: 8 in, 4 out]
  n315 = call <instrlib>:"SE Mask Offset Outer List Start Query Abs Amp Limit.vi"() -> ()  [unwired: 8 in, 4 out]
  n316 = call <instrlib>:"SE Mask Trace Fetch.vi"() -> ("instrument handle out"=w5:refnum<k15>)  [unwired: 8 in, 3 out]
  n317 = call <instrlib>:"SE Mask Offset Outer List BW Query Meas Multiplier.vi"() -> ()  [unwired: 8 in, 4 out]
  n318 = call <instrlib>:"SE Mask Offset Outer List Stop Query Abs Amp Limit Couple Enabled.vi"() -> ()  [unwired: 8 in, 4 out]
  n319 = call <instrlib>:"Read.vi"() -> ()  [unwired: 8 in, 4 out]
  n320 = call <instrlib>:"ACP Offset Outer List Filter Query Enabled.vi"() -> ()  [unwired: 8 in, 4 out]
  n321 = call <instrlib>:"Query Carrier Method.vi"() -> ()  [unwired: 8 in, 4 out]
  n322 = call <instrlib>:"ACP Offset Outer List Query Enabled.vi"() -> ()  [unwired: 8 in, 4 out]
  n323 = call <instrlib>:"SE Mask Offset Outer List Query Sideband Selection.vi"("instrument handle"=w4) -> ("instrument handle out"=w3:refnum<k15>)  [unwired: 7 in, 3 out]
  n324 = call <instrlib>:"SE Mask Offset List Query Ratio.vi"() -> ()  [unwired: 8 in, 4 out]
  n325 = call <instrlib>:"SE Mask Offset List Start Query Frequency.vi"() -> ()  [unwired: 8 in, 4 out]
  n326 = call <instrlib>:"Query Absolute Amplitude Limit Couple Enabled.vi"() -> ()  [unwired: 8 in, 4 out]
  n327 = call <instrlib>:"Query IF Gain State.vi"() -> ()  [unwired: 8 in, 4 out]
  n328 = call <instrlib>:"Query Attenuation.vi"() -> ()  [unwired: 8 in, 4 out]
  n329 = call <instrlib>:"Query Peak Threshold.vi"() -> ()  [unwired: 8 in, 4 out]
  n330 = call <instrlib>:"Spurious Emissions Range Table BW Query Resolution Auto Enabled.vi"() -> ()  [unwired: 8 in, 4 out]
  n331 = call <instrlib>:"Spurious Emissions RangeTable Start Query Frequency.vi"() -> ()  [unwired: 8 in, 4 out]
  n332 = call <instrlib>:"Query Absolute Stop Limit.vi"() -> ()  [unwired: 8 in, 4 out]
  n333 = call <instrlib>:"Waveform Trace Read.vi"() -> ()  [unwired: 8 in, 4 out]
  n334 = call <instrlib>:"ACP Offset Outer List BW Query Ref.vi"() -> ()  [unwired: 8 in, 4 out]
  n335 = call <instrlib>:"Channel Power Trace Read.vi"() -> ()  [unwired: 8 in, 4 out]
  n336 = call <instrlib>:"Digital Demod Trace Read.vi"() -> ()  [unwired: 8 in, 4 out]
  n337 = call <instrlib>:"Monitor Trace Read.vi"() -> ()  [unwired: 8 in, 4 out]
  n338 = call <instrlib>:"Occupied Bandwidth Trace Read.vi"() -> ()  [unwired: 8 in, 4 out]
  n339 = call <instrlib>:"Power Statistics Trace Read.vi"() -> ()  [unwired: 8 in, 4 out]
  n340 = call <instrlib>:"SE Mask Offset Outer List Start Query Frequency.vi"() -> ()  [unwired: 8 in, 4 out]
  n341 = call <instrlib>:"SE Mask Offset List Query Sideband Selection.vi"() -> ()  [unwired: 8 in, 4 out]
  n342 = call <instrlib>:"SE Mask Offset Outer List BW Query Ratio Auto Enabled.vi"() -> ()  [unwired: 8 in, 4 out]
  n343 = call <instrlib>:"SE Mask Offset Outer List Stop Query Abs Amp Limit.vi"() -> ()  [unwired: 8 in, 4 out]
  n344 = call <instrlib>:"SE Mask Trace Read.vi"("instrument handle"=w5) -> ()  [unwired: 7 in, 4 out]
  n345 = call <instrlib>:"Carrier Lists Query Channel Spacing.vi"() -> ()  [unwired: 8 in, 4 out]
  n346 = call <instrlib>:"SE Mask Offset Outer List Query Sweep Time Auto Enabled.vi"("instrument handle"=w3) -> ("instrument handle out"=w2:refnum<k15>)  [unwired: 7 in, 3 out]
  n347 = call <instrlib>:"ACP Offset Outer List Query Frequency.vi"() -> ()  [unwired: 8 in, 4 out]
  n348 = call <instrlib>:"ACP Offset Outer List BW Query Resolution.vi"() -> ()  [unwired: 8 in, 4 out]
  n349 = call <instrlib>:"SE Mask Offset List Stop Query Frequency.vi"() -> ()  [unwired: 8 in, 4 out]
  n350 = call <instrlib>:"Query Attenuation Enabled.vi"() -> ()  [unwired: 8 in, 4 out]
  n351 = call <instrlib>:"Query Range.vi"() -> ()  [unwired: 8 in, 4 out]
  n352 = call <instrlib>:"Spurious Emissions Range Table BW Query Shape.vi"() -> ()  [unwired: 8 in, 4 out]
  n353 = call <instrlib>:"Query Stop Frequency.vi"() -> ()  [unwired: 8 in, 4 out]
  n354 = call <instrlib>:"Query List Data.vi"() -> ()  [unwired: 8 in, 4 out]
  n355 = call <instrlib>:"SE Mask Offset Outer List BW Query Ratio.vi"() -> ()  [unwired: 8 in, 4 out]
  n356 = call <instrlib>:"SE Mask Offset Outer List Start Query Rel Amp Limit.vi"() -> ()  [unwired: 8 in, 4 out]
  n357 = call <instrlib>:"SE Mask Offset Outer List Stop Query Frequency.vi"() -> ()  [unwired: 8 in, 4 out]
  n358 = call <instrlib>:"SE Mask Offset List Query Sweep Time.vi"() -> ()  [unwired: 8 in, 4 out]
  n359 = call <instrlib>:"SE Mask Offset List Query Ratio Auto Enabled.vi"() -> ()  [unwired: 8 in, 4 out]
  n360 = call <instrlib>:"SE Mask Offset List Start Query Relative Amplitude Limit.vi"() -> ()  [unwired: 8 in, 4 out]
  n361 = call <instrlib>:"SE Mask Offset Outer List Query Sweep Time.vi"("instrument handle"=w2) -> ("instrument handle out"=w1:refnum<k15>)  [unwired: 7 in, 3 out]
  n362 = call <instrlib>:"ACP Offset Outer List Query Sideband Selection.vi"() -> ()  [unwired: 8 in, 4 out]
  n363 = call <instrlib>:"Carrier Lists Query Coupling Enabled.vi"() -> ()  [unwired: 8 in, 4 out]
  n364 = call <instrlib>:"ACP Offset Outer List BW Query Shape.vi"() -> ()  [unwired: 8 in, 4 out]
  n365 = call <instrlib>:"SE Mask Offset Outer List BW Query Resolution Auto Enabled.vi"() -> ()  [unwired: 8 in, 4 out]
  n366 = call <instrlib>:"SE Mask Offset Outer List Stop Query Rel Amp Limit Auto Enabled.vi"() -> ()  [unwired: 8 in, 4 out]
  n367 = call <instrlib>:"SE Mask Offset List Stop Query Relative Amplitude Limit.vi"() -> ()  [unwired: 8 in, 4 out]
  n368 = call <instrlib>:"Query Center Frequency.vi"() -> ()  [unwired: 8 in, 4 out]
  n369 = call <instrlib>:"Query Range Auto Enabled.vi"() -> ()  [unwired: 8 in, 4 out]
  n370 = call <instrlib>:"Range Table BW Query Video.vi"() -> ()  [unwired: 8 in, 4 out]
  n371 = call <instrlib>:"Digital Demod Trace LimitY Query List Data.vi"() -> ()  [unwired: 8 in, 4 out]
  n372 = call <instrlib>:"SE Mask Offset List Query Sweep Time Auto Enabled.vi"() -> ()  [unwired: 8 in, 4 out]
  n373 = call <instrlib>:"SE Mask Offset List Bandwidth Query Resolution.vi"() -> ()  [unwired: 8 in, 4 out]
  n374 = call <instrlib>:"SE Mask Offset Outer List Query Sweep Type Auto Enabled.vi"("instrument handle"=w1) -> ()  [unwired: 7 in, 4 out]
  n375 = call <instrlib>:"ACP Offset Outer List Query Test.vi"() -> ()  [unwired: 8 in, 4 out]
  n376 = call <instrlib>:"ACP Offset Outer List BW Query Type.vi"() -> ()  [unwired: 8 in, 4 out]
  n377 = call <instrlib>:"Query Integration Bandwidth.vi"() -> ()  [unwired: 8 in, 4 out]
  n378 = call <instrlib>:"SE Mask Offset Outer List BW Query Resolution.vi"() -> ()  [unwired: 8 in, 4 out]
  n379 = call <instrlib>:"SE Mask Offset Outer List Stop Query Rel Amp Limit.vi"() -> ()  [unwired: 8 in, 4 out]
  n380 = call <instrlib>:"SE Mask Offset List Query Sweep Type.vi"() -> ()  [unwired: 8 in, 4 out]
  n381 = call <instrlib>:"SE Mask Offset List Bandwidth Query Resolution Auto Enabled.vi"() -> ()  [unwired: 8 in, 4 out]
  n382 = call <instrlib>:"Query Relative Amplitude Limit Auto Enabled.vi"() -> ()  [unwired: 8 in, 4 out]
  n383 = call <instrlib>:"Spurious Emissions Range Table Query Detector1 Types.vi"() -> ()  [unwired: 8 in, 4 out]
  n384 = call <instrlib>:"Query Sweep Points.vi"() -> ()  [unwired: 8 in, 4 out]
  n385 = call <instrlib>:"Range Table BW Query Video Auto Enabled.vi"() -> ()  [unwired: 8 in, 4 out]
  n386 = call <instrlib>:"SE Mask Offset Outer List Query Sweep Type.vi"() -> ()  [unwired: 8 in, 4 out]
  n387 = call <instrlib>:"ACP Offset Outer List Query Relative Limit Carrier.vi"() -> ()  [unwired: 8 in, 4 out]
  n388 = call <instrlib>:"ACP Offset Outer List BW Query Video Auto Enabled.vi"() -> ()  [unwired: 8 in, 4 out]
  n389 = call <instrlib>:"SE Mask Offset Outer List BW Query Video Auto Enabled.vi"() -> ()  [unwired: 8 in, 4 out]
  n390 = call <instrlib>:"Query Method Types.vi"() -> ()  [unwired: 8 in, 4 out]
  n391 = call <instrlib>:"Query Measurement Multiplier.vi"() -> ()  [unwired: 8 in, 4 out]
  n392 = call <instrlib>:"SE Mask Offset List Query Sweep Type Auto Enabled.vi"() -> ()  [unwired: 8 in, 4 out]
  n393 = call <instrlib>:"SE Mask Offset List BW Query Video Auto Enabled.vi"() -> ()  [unwired: 8 in, 4 out]
  n394 = call <instrlib>:"Spurious Emissions Range Table Query Detector2 Types.vi"() -> ()  [unwired: 8 in, 4 out]
  n395 = call <instrlib>:"Query Sweep Points Auto Enabled.vi"() -> ()  [unwired: 8 in, 4 out]
  n396 = call <instrlib>:"SE Mask Offset Outer List Query Test.vi"() -> ()  [unwired: 8 in, 4 out]
  n397 = call <instrlib>:"ACP Offset Outer List Query Relative Limit PSD.vi"() -> ()  [unwired: 8 in, 4 out]
  n398 = call <instrlib>:"ACP Offset Outer List BW Query Video.vi"() -> ()  [unwired: 8 in, 4 out]
  n399 = call <instrlib>:"SE Mask Offset Outer List BW Query Video.vi"() -> ()  [unwired: 8 in, 4 out]
  n400 = call <instrlib>:"Query Power Present.vi"() -> ()  [unwired: 8 in, 4 out]
  n401 = call <instrlib>:"SE Mask Offset List Query Test.vi"() -> ()  [unwired: 8 in, 4 out]
  n402 = call <instrlib>:"Spurious Emissions Range Table Query Enabled.vi"() -> ()  [unwired: 8 in, 4 out]
  n403 = call <instrlib>:"Spurious Emissions Range Table Query Sweep Time Auto Enabled.vi"() -> ()  [unwired: 8 in, 4 out]
  n404 = call <instrlib>:"Query SweepTime.vi"() -> ()  [unwired: 8 in, 4 out]
  n405 = call <instrlib>:"Disable.vi"() -> ()  [unwired: 10 in, 2 out]
  n406 = call <instrlib>:"Error Message.vi"() -> ()  [unwired: 9 in, 3 out]
  n407 = call <instrlib>:"Error-Query.vi"() -> ()  [unwired: 8 in, 4 out]
  n408 = call <instrlib>:"Reset.vi"() -> ()  [unwired: 10 in, 2 out]
  n409 = call <instrlib>:"Reset With Defaults.vi"() -> ()  [unwired: 10 in, 2 out]
  n410 = call <instrlib>:"Revision Query.vi"() -> ()  [unwired: 8 in, 4 out]
  n411 = call <instrlib>:"Self-Test.vi"() -> ()  [unwired: 8 in, 4 out]
  n412 = call <instrlib>:"Close.vi"() -> ()  [unwired: 11 in, 1 out]
